vi "roboRIO Name Align Center.vi"(8 "error in (no error)":errorcluster, 10 "Target Refnum":refnum<vi>, 11 "Ref Control":refnum<vi>) -> (0 "error out":errorcluster)   [LabVIEW 2021]
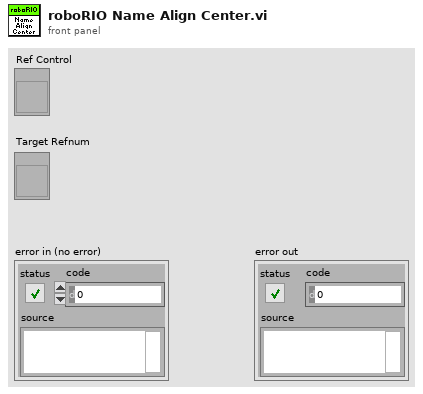
[diagram p1: front panel]
types:
  T1 = cluster{"Font Name:":string, "Size":i16, "Strikeout?":bool, "Italic?":bool, "Underline?":bool, "Outline?":bool, "Shadow?":bool, "Bold?":bool}
  T2 = enum16{"User-specified Font", "Application Font", "System Font", "Dialog Font"}
  T3 = typedef "LVFontTypeDef.ctl" = cluster{"Font Name":string, "Size":u16, "Bold":bool, "Italic":bool, "Underline":bool, "Strikeout":bool, "Color":u32}
  T4 = cluster{"left":i16, "top":i16, "right":i16, "bottom":i16}
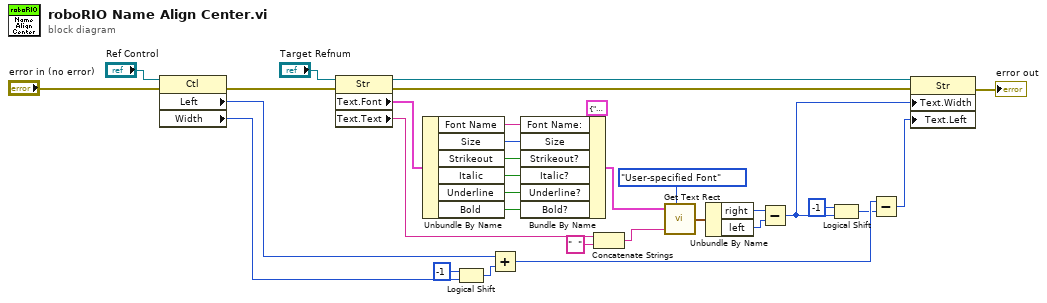
[diagram p0: block diagram]
diagram:
  n1 = property class="Ctl"(reference="Ref Control", error in="error in (no error)") -> (error out=w5:errorcluster, "Left"=w27:i32, "Width"=w30:u32)  [unwired: 1 out]
  n2 = property class="Str"(reference="Target Refnum", error in=w5) -> (reference out=w26:refnum<vi>, error out=w32:errorcluster, "Text.Font"=w12:T3, "Text.Text"=w10:string)
  n3 = Unbundle By Name(w12) -> ("Font Name"=w23:string, "Size"=w22:u16, "Strikeout"=w21:bool, "Italic"=w20:bool, "Underline"=w19:bool, "Bold"=w18:bool)
  n4 = Logical Shift(y=i16 -1, x=w30) -> (x << y=w28:u32)
  n5 = Add(x=w27, y=w28) -> (x+y=w25:u32)
  n6 = Bundle By Name(cluster=T1 {"Font Name:"="", "Size"=0, "Strikeout?"=FALSE, "Italic?"=FALSE, "Underline?"=FALSE, "Outline?"=FALSE, "Shadow?"=FALSE, "Bold?"=FALSE} ("Font Info"), "Font Name:"=w23, "Size"=w22, "Strikeout?"=w21, "Italic?"=w20, "Underline?"=w19, "Bold?"=w18) -> (w16:T1)
  n7 = Concatenate Strings(w10, "  " ("string")) -> (w11:string)
  n8 = call <vilib>:"Get Text Rect.vi"("desired font(Application)"=T2."User-specified Font", "text"=w11, "[user-specified font]"=w16) -> ("rect"=w13:T4)  [unwired: 6 in]
  n9 = Unbundle By Name(w13) -> ("right"=w14:i16, "left"=w15:i16)
  n10 = Subtract(x=w14, y=w15) -> (x-y=w2:i16)
  n11 = Logical Shift(y=i16 -1, x=w2) -> (x << y=w7:i16)
  n12 = Subtract(x=w25, y=w7) -> (x-y=w1:u32)
  n13 = property class="Str"(reference=w26, error in=w32, "Text.Width"=w2, "Text.Left"=w1) -> (error out=→"error out":errorcluster)  [unwired: 1 out]
